vi "Read (Single Point).vi"(0 "VISA resource name":refnum<visa-resource-name>, 5 "Timeout (10000 ms)":i32=10000 format="%#.6g", 11 "error in (no error)":errorcluster) -> (3 "Voltage":sgl, 4 "VISA resource name out":refnum<visa-resource-name>, 6 "Current":sgl, 8 "Resistance":sgl, 10 "Timestamp":sgl, 14 "Status":sgl, 15 "error out":errorcluster)   [LabVIEW 2012, in "Keithley 24XX.lvlib"]
doc: "Reads and returns a single measurement from the instrument.\n\n<B>Note:</B> Using this VI will overwrite all triggering settings with settings for a single point taken immediately. For control over the trigger, use the Low Level API."
uses:
  Keithley 24XX.lvlib
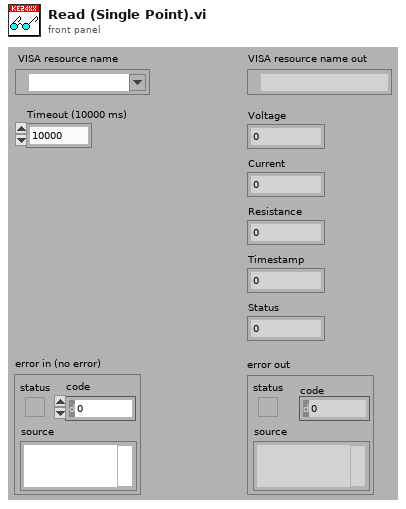
[diagram p1: front panel]
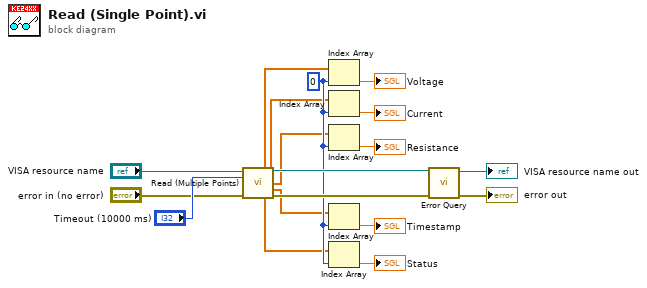
[diagram p0: block diagram]
diagram:
  w14 = 0 ("index")
  n1 = call "Read (Multiple Points).vi"("VISA resource name"="VISA resource name", "Timeout (10000 ms)"="Timeout (10000 ms)", "error in (no error)"="error in (no error)") -> ("Voltage"=w13:sgl[], "VISA resource name out"=w15:refnum<visa-resource-name>, "Current"=w12:sgl[], "Resistance"=w11:sgl[], "Timestamp"=w10:sgl[], "Status"=w9:sgl[], "error out"=w16:errorcluster)  [unwired: 6 in]
  n2 = Index Array(array=w13, index=w14) -> (element=→"Voltage":sgl)
  n3 = Index Array(array=w12, index=w14) -> (element=→"Current":sgl)
  n4 = Index Array(array=w11, index=w14) -> (element=→"Resistance":sgl)
  n5 = Index Array(array=w10, index=w14) -> (element=→"Timestamp":sgl)
  n6 = Index Array(array=w9, index=w14) -> (element=→"Status":sgl)
  n7 = call "Error Query.vi"("error in (no error)"=w16, "VISA resource name"=w15) -> ("error out"=→"error out":errorcluster, "VISA resource name out"=→"VISA resource name out":refnum<visa-resource-name>)  [unwired: 6 in, 2 out]
